vi "TTA_MATLAB_Tile_RFPAL_Load_Cal_SetClear.vi"(0 "Channels":string[](array[combo]), 5 "Mode":string(combo)="Clear", 7 "Frequency":dbl, 11 "error in":errorcluster) -> (4 "Success":bool, 6 "TileSuccessOp":bool[](array[boolean]), 8 "TileSuccessComm":bool[](array[boolean]), 15 "error out":errorcluster)   [LabVIEW 2016]
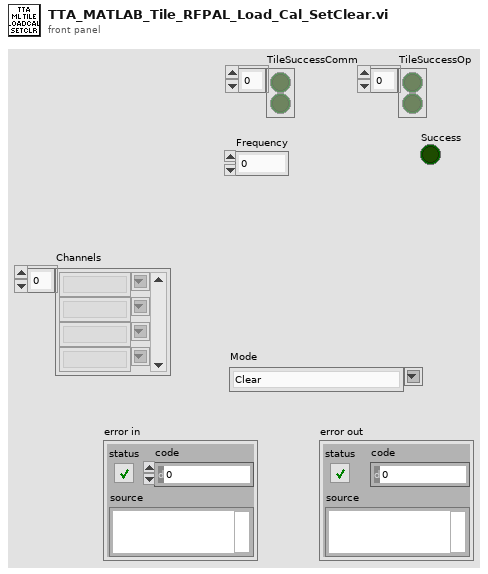
[diagram p1: front panel]
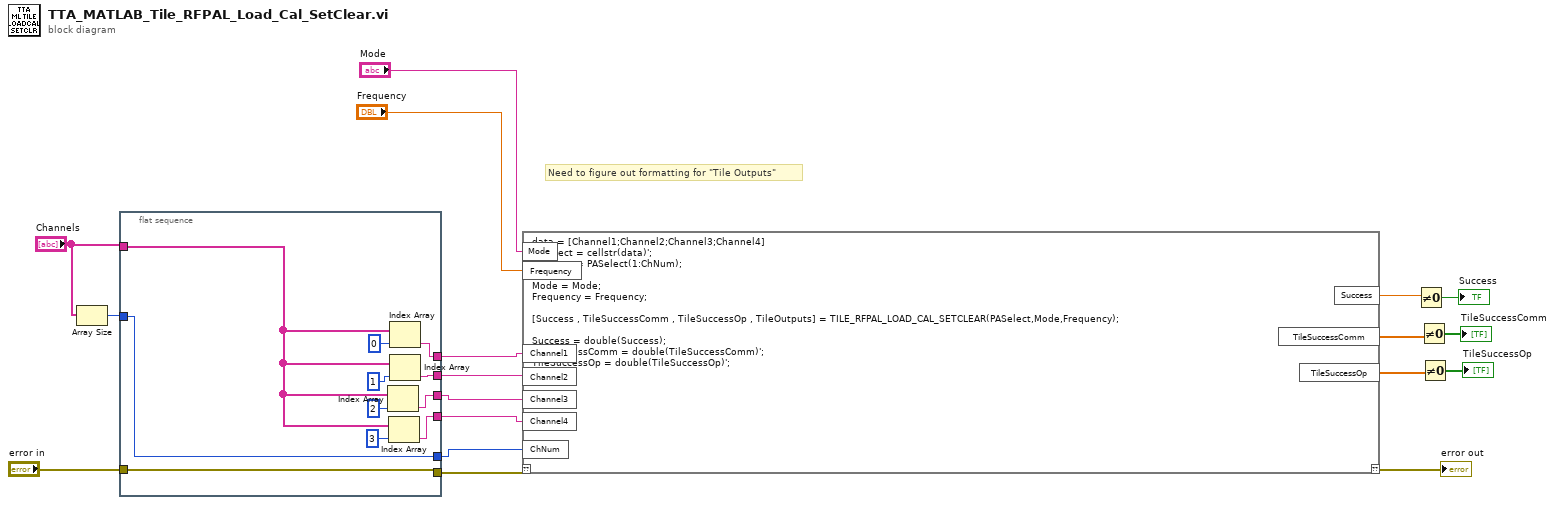
[diagram p0: block diagram]
diagram:
  # "Need to figure out formatting for \"Tile Outputs\""
  n1 = Array Size(array="Channels") -> (size(s)=w6:i32)
  n2 = flat-sequence {
    tunnel: "error in" -> [w29]
    tunnel: [w28] -> w5
    tunnel: w6 -> [w22]
    tunnel: [w29] -> w8
    tunnel: "Channels" -> [w21]
    tunnel: [w25] -> w4
    tunnel: [w23] -> w3
    tunnel: [w22] -> w1
    tunnel: [w19] -> w2
    frame #0 {
      n3 = Index Array(array=w21, index=2) -> (element=w23:string)
      n4 = Index Array(array=w21, index=3) -> (element=w19:string)
      n5 = Index Array(array=w21, index=0) -> (element=w28:string)
      n6 = Index Array(array=w21, index=1) -> (element=w25:string)
    }
  }
  n7 = script code="data = [Channel1;Channel2;Channel3;Channel4]\nPASelect = cellstr(data)';\nPASelect = PASelect(1:ChNum);\n\nMode = Mode;\nFrequency = Frequency;\n\n[Success , TileSuccessComm , TileSuccessOp , TileOutputs] = TILE_RFPAL_LOAD_CAL_SETCLEAR(PASelect,Mode,Frequency);\n\nSuccess = double(Success);\nTileSuccessComm = double(TileSuccessComm)';\nTileSuccessOp = double(TileSuccessOp)';"("??"=w8, "Channel1"=w5, "Mode"="Mode", "Frequency"="Frequency", "Channel2"=w4, "Channel3"=w3, "Channel4"=w2, "ChNum"=w1) -> ("??"=→"error out":errorcluster, "Success"=w13:dbl, "TileSuccessComm"=w12:dbl[], "TileSuccessOp"=w11:dbl[])
  n8 = Not Equal To 0?(x=w13) -> (x != 0?=→"Success":bool)
  n9 = Not Equal To 0?(x=w12) -> (x != 0?=→"TileSuccessComm":bool[])
  n10 = Not Equal To 0?(x=w11) -> (x != 0?=→"TileSuccessOp":bool[])
